vi "ChannelSettings.vi"() -> ()   [LabVIEW 2019]
uses:
  <vilib>/Bytelabs/ByteChannelsSetting/ChannelSettingsLib/ChannelsClasses/ChannelAnalog/AnalogRio/AnalogRio.lvclass
  C:/Program Files (x86)/National Instruments/LabVIEW 2019/vi.lib/Bytelabs/ByteChannelsSetting/ChannelSettingsLib/ChannelsClasses/ChannelAnalog/AnalogIn/AnalogIn.lvclass
  TypeDef/SubPanelType.ctl
  <vilib>/Bytelabs/ByteChannelsSetting/ChannelSettingsLib/ChannelsRepos/ChannelsRepoXML/ChannelsRepoXML.lvclass
  C:/Program Files (x86)/National Instruments/LabVIEW 2019/vi.lib/Bytelabs/ByteChannelsSetting/ChannelSettingsLib/ChannelsRepos/ChannelsRepoBase/ChannelsRepoBase.lvclass
  <vilib>/Bytelabs/ByteChannelsSetting/ChannelSettingsLib/ChannelsRepos/ChannelsRepoBase/ShowCreateUI.vi
  <vilib>/Bytelabs/ByteChannelsSetting/ChannelSettingsLib/ChannelsRepos/ChannelsRepoBase/ShowChannelConfiguration.vi
  <vilib>/Bytelabs/ByteChannelsSetting/ChannelSettingsLib/ChannelsRepos/ChannelsRepoBase/ChannelsRepoBase.lvclass
  <vilib>/Bytelabs/ByteSimpleQ/ByteSimpleQ/ByteSimpleQ.lvlib
panel:
  in  "Tree":string(tree)
  in  "Create":bool caption="Add Row"
  in  "Delete":bool caption="Delete Row"
  in  "Exit":bool
  in  "Apply":bool
  # "CHANNEL SETTING"
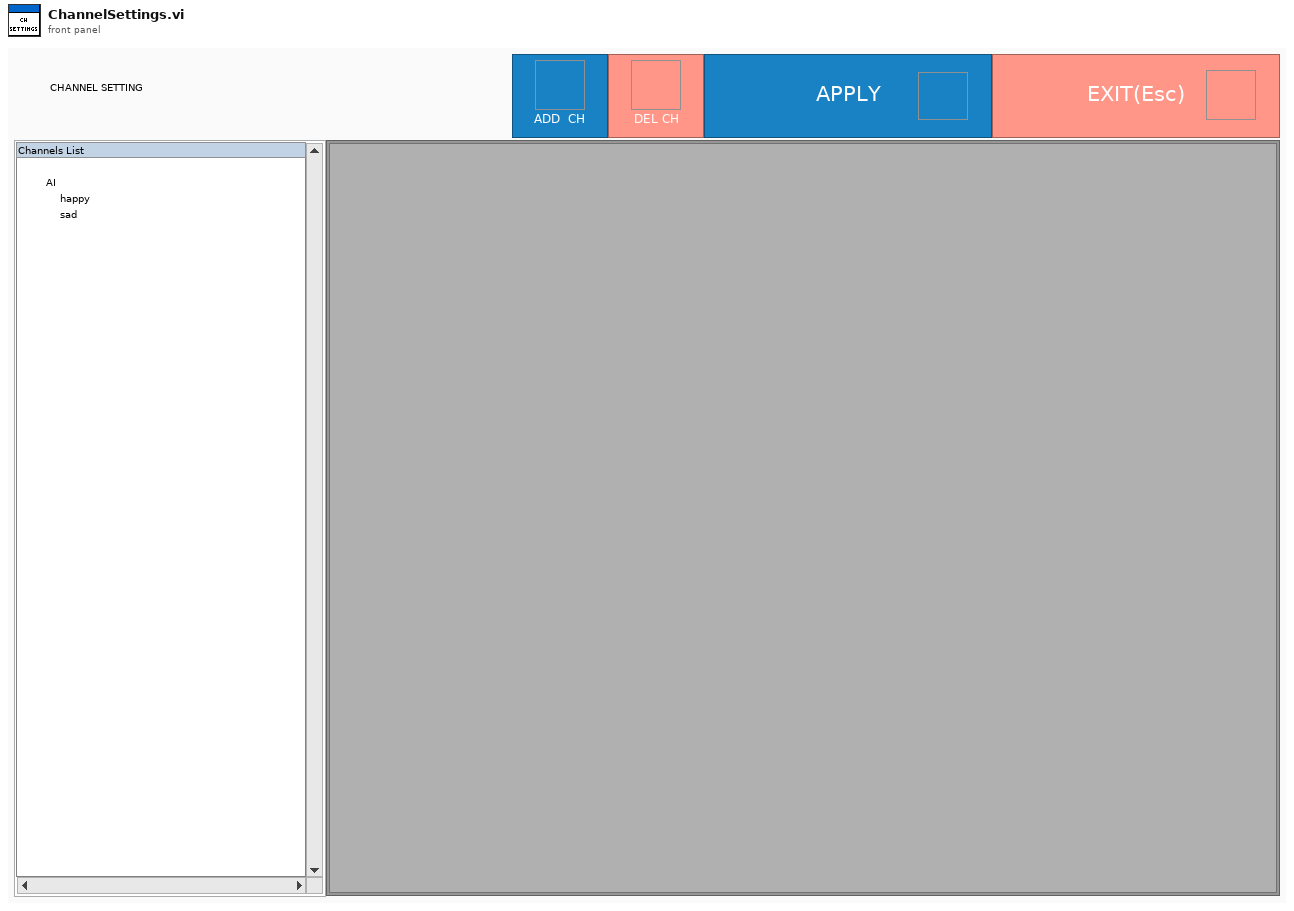
[diagram p1: front panel]
types:
  T1 = enum8{"Enabled", "Disabled", "Disabled and Grayed Out"}
  T2 = cluster{"queue out":refnum<queue>, "ChannelsRepoBase out":refnum<class "ChannelsRepoXML.lvclass">, "Close Event":refnum<user-event>, "Modify Ref":refnum<vi>, "Create Ref":refnum<vi>, "Mode":string, "Tree":refnum<vi>, "Tag":string, "ChannelsRepoBase out":refnum<class "ChannelsRepoXML.lvclass">}
  T3 = typedef "SubPanelType.ctl" = cluster{"Modality":string, "Tag":string}
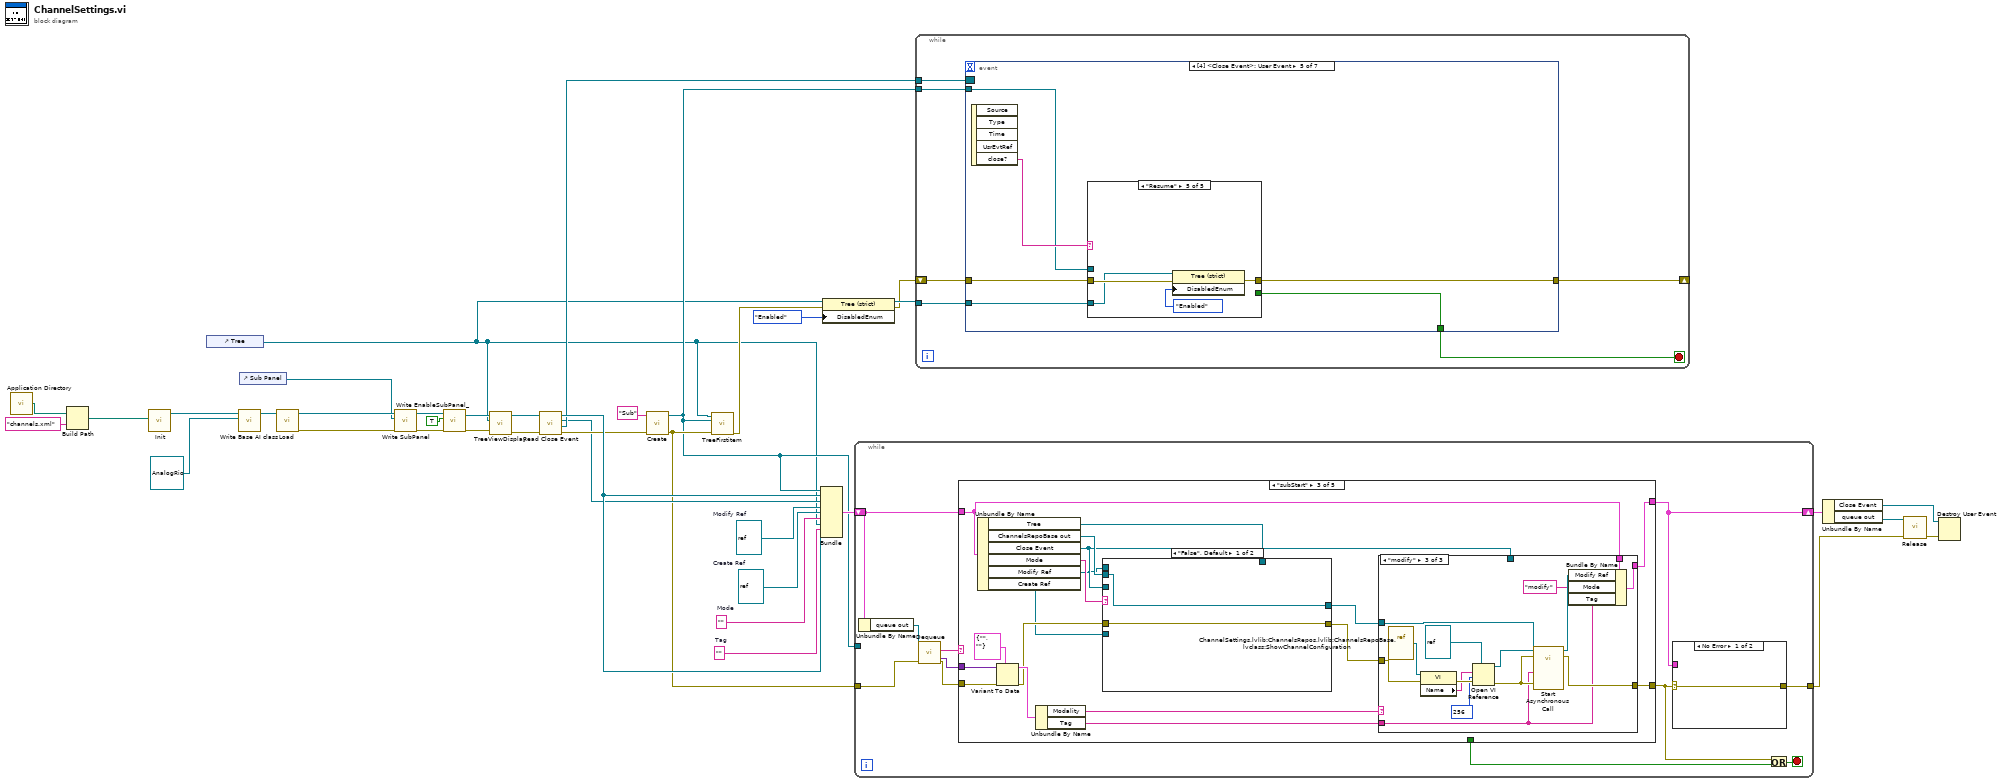
[diagram p0: block diagram]
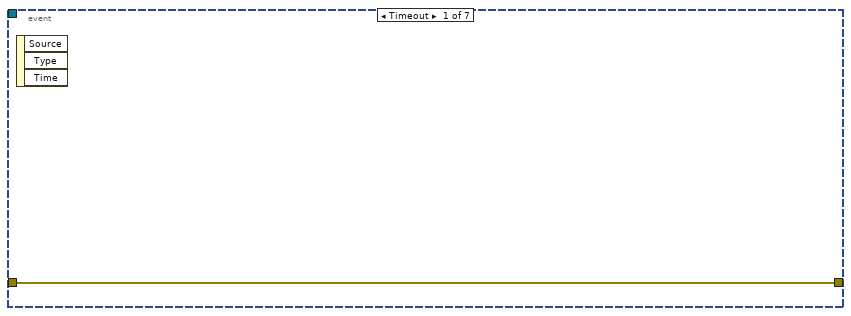
[diagram p2: hidden frame]
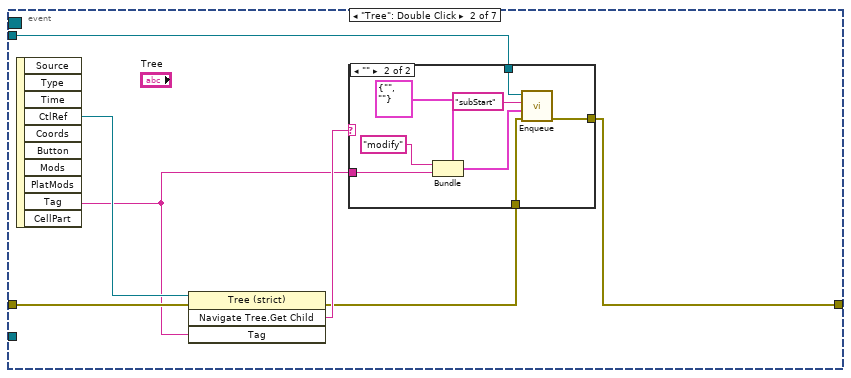
[diagram p3: hidden frame]
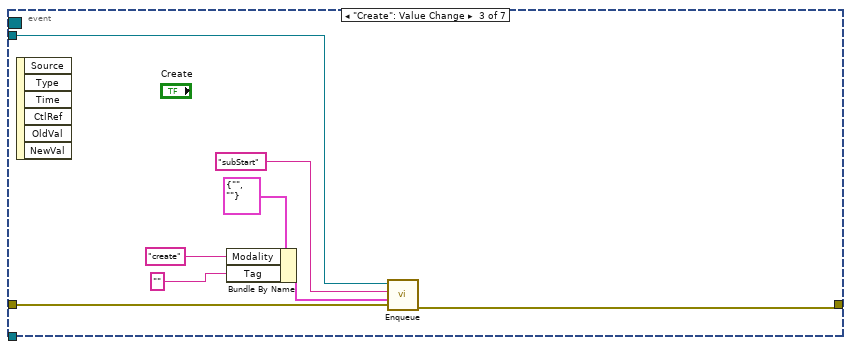
[diagram p5: hidden frame]
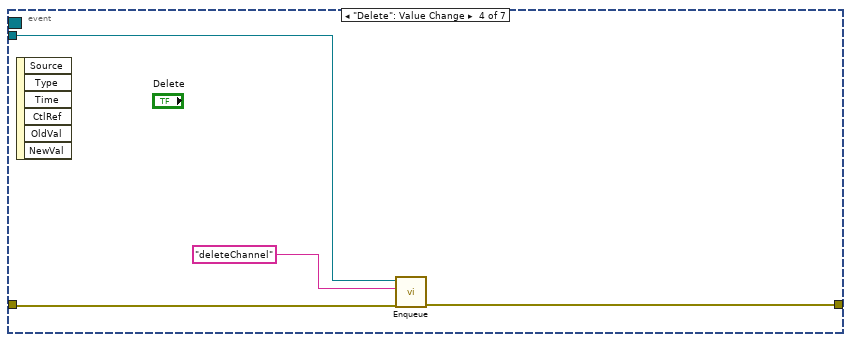
[diagram p6: hidden frame]
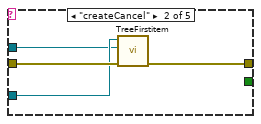
[diagram p8: hidden frame]
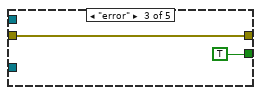
[diagram p9: hidden frame]
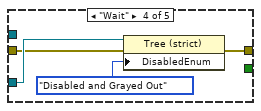
[diagram p10: hidden frame]
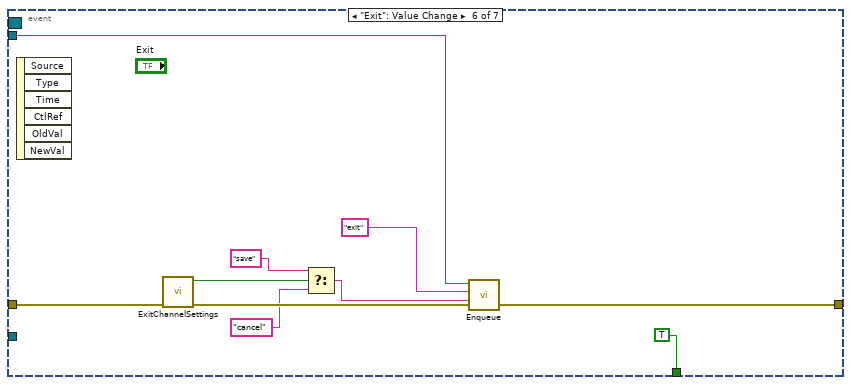
[diagram p11: hidden frame]
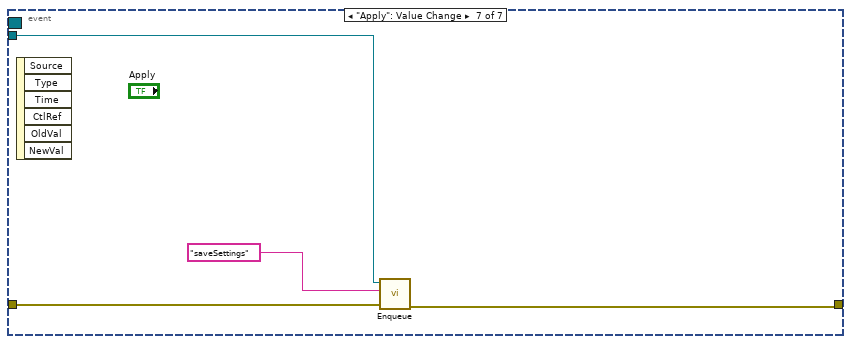
[diagram p12: hidden frame]
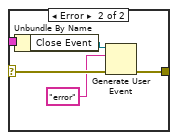
[diagram p13: hidden frame]
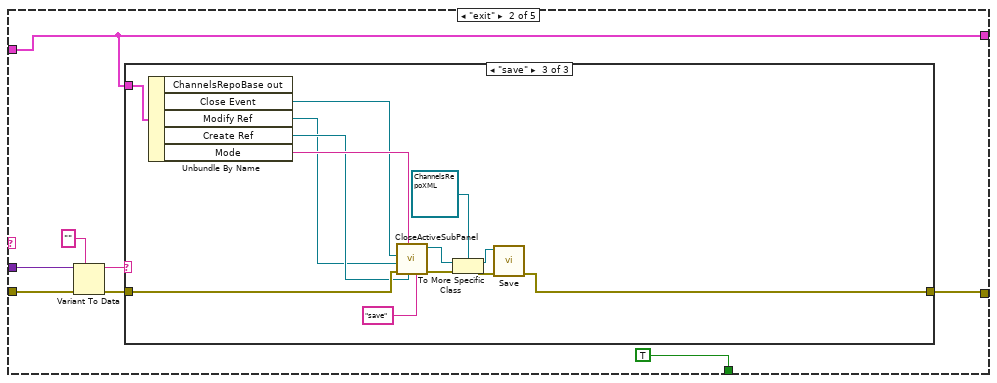
[diagram p15: hidden frame]
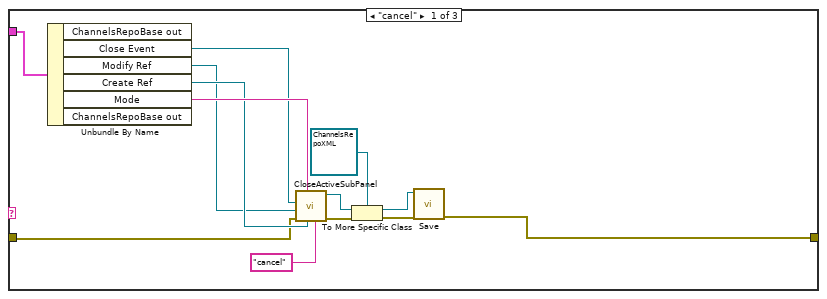
[diagram p16: hidden frame]
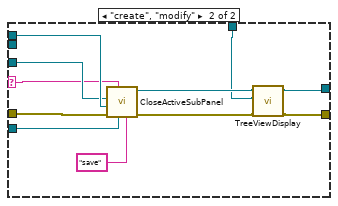
[diagram p18: hidden frame]
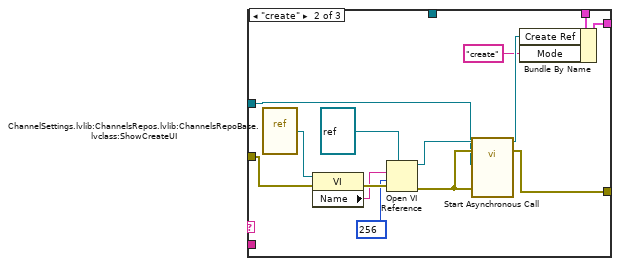
[diagram p20: hidden frame]
diagram:
  w29 = ""  # Tag
  w33 = refnum<vi> refnum  # Create Ref
  w34 = refnum<vi> refnum  # Modify Ref
  w32 = ""  # Mode
  n1 = call <vilib>:"Application Directory.vi"() -> ("Application Directory"=w18:path)
  n2 = Build Path(base path=w18, name or relative path="channels.xml") -> (appended path=w16:path)
  n3 = call <vilib>:"Init.vi"("XML file path"=w16) -> ("ChannelsRepoXML out"=w17:refnum<class "ChannelsRepoXML.lvclass">)  [unwired: 10 in]
  n4 = control-ref of="Tree"() -> (w5:refnum<vi>)
  n5 = call-dynamic "Write Base AI class.vi"("ChannelsClasses.lvlib:AnalogIn.lvclass"=refnum<class "AnalogRio.lvclass"> refnum ("ChannelSettings.lvlib:ChannelsClasses.lvlib:AnalogRio.lvclass"), "ChannelsRepoBase in"=w17) -> ("ChannelsRepoBase out"=w11:refnum<class "ChannelsRepoXML.lvclass">)  [unwired: 9 in]
  n6 = control-ref of="Sub Panel"() -> (w1:refnum<vi>)
  n7 = call <vilib>:"Load.vi"("ChannelsRepoBase in"=w11) -> ("error out"=w3:errorcluster, "ChannelsRepoBase out"=w35:refnum<class "ChannelsRepoXML.lvclass">)  [unwired: 8 in, 1 out]
  n8 = call-dynamic "Write SubPanel.vi"("error in (no error)"=w3, "SubPanel"=w1, "ChannelsRepoBase in"=w35) -> ("error out"=w38:errorcluster, "ChannelsRepoBase out"=w37:refnum<class "ChannelsRepoXML.lvclass">)  [unwired: 7 in]
  n9 = call-dynamic "Write EnableSubPanel_.vi"("error in (no error)"=w38, "EnableSubPanel?"=TRUE, "ChannelsRepoBase in"=w37) -> ("error out"=w15:errorcluster, "ChannelsRepoBase out"=w12:refnum<class "ChannelsRepoXML.lvclass">)  [unwired: 7 in]
  n10 = call-dynamic "TreeViewDisplay.vi"("error in (no error)"=w15, "Tree ref"=w5, "ChannelsRepoBase in"=w12) -> ("error out"=w14:errorcluster, "ChannelsRepoBase out"=w13:refnum<class "ChannelsRepoXML.lvclass">)  [unwired: 7 in]
  n11 = call-dynamic "Read Close Event.vi"("error in (no error)"=w14, "ChannelsRepoBase in"=w13) -> ("error out"=w22:errorcluster, "Event Refnum"=w21:refnum<event-registration>, "Close Event"=w20:refnum<user-event>, "ChannelsRepoBase out"=w23:refnum<class "ChannelsRepoXML.lvclass">)  [unwired: 6 in]
  n12 = call <vilib>:"Create.vi"("error in (no error)"=w22, "name (unnamed)"="Sub") -> ("error out"=w10:errorcluster, "queue out"=w9:refnum<queue>)  [unwired: 7 in, 1 out]
  n13 = call <vilib>:"TreeFirstitem.vi"("error in (no error)"=w10, "queue in"=w9, "TreeControl in"=w5) -> ("error out"=w7:errorcluster)  [unwired: 8 in]
  n14 = Bundle("queue out"=w9, "ChannelsRepoBase out"=w23, "Close Event"=w20, "Modify Ref"=w34, "Create Ref"=w33, "Mode"=w32, "Tree"=w5, "Tag"=w29, "ChannelsRepoBase out"=w23) -> (w31:T2)  [unwired: 1 in]
  n15 = property class="Tree (strict)"(reference=w5, error in=w7, "DisabledEnum"=T1."Enabled" ("Disabled")) -> (reference out=w6:refnum<vi>, error out=w4:errorcluster)
  n16 = while {
    tunnel: w9 -> [_]
    shift-right: [w41] -> w28
    shift-left: w31 -> [w40]
    tunnel: w10 -> [w49]
    tunnel: [w45] -> w26
    stop <- w44 stop-if-true
    n17 = Unbundle By Name(w40) -> ("queue out"=w39:refnum<queue>)
    n18 = call <vilib>:"Dequeue.vi"("error in (no error)"=w49, "queue in"=w39) -> ("error out"=w46:errorcluster, "data"=w47:variant, "message"=w48:string)  [unwired: 5 in, 2 out]
    n19 = case shown="\"subStart\"" w48 {
      tunnel: w47 -> [_ w63 w109 _ _]
      tunnel: w46 -> [w57 w64 w110 w166 w219]
      tunnel: w40 -> [w56 w58 w108 w157 w220]
      tunnel: [w57 w59 w106 w164 w213] -> w42
      tunnel: [w56 w58 w107 w156 w212] -> w41
      tunnel: [_ TRUE _ _ _] -> w43
      frame Default {
      }
      frame "exit" {
        n20 = Variant To Data(error in=w64, type="" ("message"), Variant=w63) -> (data=w61:string, error out=w60:errorcluster)
        n21 = case shown="\"save\"" w61 {
          tunnel: w60 -> [w70 w79 w88]
          tunnel: [w67 w79 w81] -> w59
          tunnel: w58 -> [w71 _ w89]
          frame "cancel" {
            n22 = Unbundle By Name(w71) -> ("Close Event"=w74:refnum<user-event>, "Modify Ref"=w72:refnum<vi>, "Create Ref"=w73:refnum<vi>, "Mode"=w75:string)  [unwired: 2 out]
            n23 = call <vilib>:"CloseActiveSubPanel.vi"("Save?"="cancel", "Create Ref"=w73, "Mode"=w75, "error in (no error)"=w70, "Modify Ref"=w72, "close?"=w74) -> ("error out"=w77:errorcluster, "ChannelsRepoBase out"=w76:refnum<class "ChannelsRepoXML.lvclass">)  [unwired: 3 in, 1 out]
            n24 = To More Specific Class(target class=refnum<class "ChannelsRepoXML.lvclass"> refnum ("ChannelsRepoBase out"), reference=w76, error in=w77) -> (specific class reference=w66:refnum<class "ChannelsRepoXML.lvclass">, error out=w68:errorcluster)
            n25 = call-dynamic "Save.vi"("error in (no error)"=w68, "ChannelsRepoXML in"=w66) -> ("error out"=w67:errorcluster)  [unwired: 8 in, 1 out]
          }
          frame Default {
          }
          frame "save" {
            n26 = Unbundle By Name(w89) -> ("Close Event"=w86:refnum<user-event>, "Modify Ref"=w84:refnum<vi>, "Create Ref"=w85:refnum<vi>, "Mode"=w87:string)  [unwired: 1 out]
            n27 = call <vilib>:"CloseActiveSubPanel.vi"("Save?"="save", "Create Ref"=w85, "Mode"=w87, "error in (no error)"=w88, "Modify Ref"=w84, "close?"=w86) -> ("error out"=w91:errorcluster, "ChannelsRepoBase out"=w90:refnum<class "ChannelsRepoXML.lvclass">)  [unwired: 3 in, 1 out]
            n28 = To More Specific Class(target class=refnum<class "ChannelsRepoXML.lvclass"> refnum ("ChannelsRepoBase out"), reference=w90, error in=w91) -> (specific class reference=w80:refnum<class "ChannelsRepoXML.lvclass">, error out=w82:errorcluster)
            n29 = call-dynamic "Save.vi"("error in (no error)"=w82, "ChannelsRepoXML in"=w80) -> ("error out"=w81:errorcluster)  [unwired: 8 in, 1 out]
          }
        }
      }
      frame "subStart" {
        n30 = Unbundle By Name(w108) -> ("Tree"=w93:refnum<vi>, "ChannelsRepoBase out"=w99:refnum<class "ChannelsRepoXML.lvclass">, "Close Event"=w97:refnum<user-event>, "Mode"=w100:string, "Modify Ref"=w96:refnum<vi>, "Create Ref"=w95:refnum<vi>)
        n31 = Variant To Data(error in=w110, type=T3 {"Modality"="", "Tag"=""}, Variant=w109) -> (data=w105:T3, error out=w103:errorcluster)
        n32 = Unbundle By Name(w105) -> ("Modality"=w94:string, "Tag"=w102:string)
        n33 = case shown="\"False\", Default" w100 {
          selector: w100 -> [_ w118]
          tunnel: w103 -> [w112 w123]
          tunnel: [w112 w114] -> w101
          tunnel: w99 -> [w111 _]
          tunnel: [w111 w117] -> w98
          tunnel: w97 -> [_ w119]
          tunnel: w96 -> [_ w120]
          tunnel: w95 -> [_ w121]
          tunnel: w93 -> [_ w113]
          frame "False", Default {
          }
          frame "create", "modify" {
            n34 = call <vilib>:"CloseActiveSubPanel.vi"("Save?"="save", "Create Ref"=w121, "Mode"=w118, "error in (no error)"=w123, "Modify Ref"=w120, "close?"=w119) -> ("error out"=w115:errorcluster, "ChannelsRepoBase out"=w116:refnum<class "ChannelsRepoXML.lvclass">)  [unwired: 3 in, 1 out]
            n35 = call-dynamic "TreeViewDisplay.vi"("error in (no error)"=w115, "Tree ref"=w113, "ChannelsRepoBase in"=w116) -> ("error out"=w114:errorcluster, "ChannelsRepoBase out"=w117:refnum<class "ChannelsRepoXML.lvclass">)  [unwired: 7 in]
          }
        }
        n36 = case shown="\"modify\"" w94 {
          tunnel: w108 -> [w124 w130 w147]
          tunnel: [w124 w129 w144] -> w107
          tunnel: [w125 w128 w143] -> w106
          tunnel: w97 -> [_ _ _]
          tunnel: w101 -> [w125 w127 w142]
          tunnel: w98 -> [_ w126 w140]
          tunnel: w102 -> [_ _ w141]
          frame Default {
          }
          frame "create" {
            n37 = vi-ref "ChannelSettings.lvlib:ChannelsRepos.lvlib:ChannelsRepoBase.lvclass:ShowCreateUI.vi"() -> (w139:refnum<vi>)
            n38 = property class="VI"(reference=w139, error in=w127) -> (error out=w138:errorcluster, "Name"=w137:string)  [unwired: 1 out]
            n39 = Open VI Reference(type specifier VI Refnum (for type only)=refnum<vi> refnum, vi path=w137, options=256, error in (no error)=w138) -> (vi reference=w134:refnum<vi>, error out=w133:errorcluster)  [unwired: 2 in]
            n40 = call-by-ref "Start Asynchronous Call"(reference=w134, error in=w133, 8:"error in (no error)"=w133, "ChannelBase in"=w126) -> (reference out=w132:refnum<vi>, error out=w128:errorcluster)  [unwired: 7 in, 3 out]
            n41 = Bundle By Name(cluster=w130, "Create Ref"=w132, "Mode"="create") -> (w129:T2)
          }
          frame "modify" {
            n42 = vi-ref "ChannelSettings.lvlib:ChannelsRepos.lvlib:ChannelsRepoBase.lvclass:ShowChannelConfiguration.vi"() -> (w154:refnum<vi>)
            n43 = property class="VI"(reference=w154, error in=w142) -> (error out=w153:errorcluster, "Name"=w152:string)  [unwired: 1 out]
            n44 = Open VI Reference(type specifier VI Refnum (for type only)=refnum<vi> refnum, vi path=w152, options=256, error in (no error)=w153) -> (vi reference=w149:refnum<vi>, error out=w148:errorcluster)  [unwired: 2 in]
            n45 = call-by-ref "Start Asynchronous Call"(reference=w149, error in=w148, 8:"error in (no error)"=w148, "tag"=w141, "ChannelsRepoBase in"=w140) -> (reference out=w146:refnum<vi>, error out=w143:errorcluster)  [unwired: 6 in, 3 out]
            n46 = Bundle By Name(cluster=w147, "Modify Ref"=w146, "Mode"="modify", "Tag"=w141) -> (w144:T2)
          }
        }
      }
      frame "deleteChannel" {
        n47 = Unbundle By Name(w157) -> ("queue out"=w155:refnum<queue>, "ChannelsRepoBase out"=w167:refnum<class "ChannelsRepoXML.lvclass">, "Close Event"=w165:refnum<user-event>, "Mode"=w161:string, "Modify Ref"=w160:refnum<vi>, "Create Ref"=w159:refnum<vi>, "Tree"=w158:refnum<vi>)  [unwired: 1 out]
        n48 = call <vilib>:"DeleteChannelConfirmation.vi"("error in (no error)"=w166) -> ("error out"=w162:errorcluster, "Confirmed"=w163:bool)  [unwired: 9 in]
        n49 = case shown="True" w163 {
          tunnel: w167 -> [_ _]
          tunnel: w165 -> [_ w186]
          tunnel: [w169 w179] -> w164
          tunnel: w162 -> [w169 w190]
          tunnel: w161 -> [_ w189]
          tunnel: w160 -> [_ w188]
          tunnel: w159 -> [_ w187]
          tunnel: w158 -> [_ w170]
          tunnel: w157 -> [w168 w183]
          tunnel: [w168 w182] -> w156
          tunnel: w155 -> [_ w178]
          frame False {
          }
          frame True {
            n50 = call <vilib>:"CloseActiveSubPanel.vi"("Save?"="cancel", "Create Ref"=w187, "Mode"=w189, "error in (no error)"=w190, "Modify Ref"=w188, "close?"=w186) -> ("error out"=w191:errorcluster, "Tag"=w184:string, "ChannelsRepoBase out"=w175:refnum<class "ChannelsRepoXML.lvclass">)  [unwired: 3 in]
            n51 = call <vilib>:"DeleteChannel.vi"("error in (no error)"=w191, "tag"=w184, "ChannelsRepoBase in"=w175) -> ("error out"=w173:errorcluster, "ChannelsRepoBase out"=w174:refnum<class "ChannelsRepoXML.lvclass">)  [unwired: 6 in, 1 out]
            n52 = call-dynamic "TreeViewDisplay.vi"("error in (no error)"=w173, "Tree ref"=w170, "ChannelsRepoBase in"=w174) -> ("error out"=w172:errorcluster, "ChannelsRepoBase out"=w171:refnum<class "ChannelsRepoXML.lvclass">)  [unwired: 7 in]
            n53 = To More Specific Class(target class=refnum<class "ChannelsRepoXML.lvclass"> refnum ("ChannelsRepoBase out"), reference=w171, error in=w172) -> (specific class reference=w177:refnum<class "ChannelsRepoXML.lvclass">, error out=w180:errorcluster)
            n54 = call <vilib>:"TreeFirstitem.vi"("error in (no error)"=w180, "queue in"=w178, "TreeControl in"=w170) -> ("error out"=w179:errorcluster)  [unwired: 8 in]
            n55 = Bundle By Name(cluster=w183, "ChannelsRepoBase out"=w177, "Mode"="") -> (w182:T2)
          }
        }
      }
      frame "saveSettings" {
        n56 = Unbundle By Name(w220) -> ("Tree"=w194:refnum<vi>, "Close Event"=w198:refnum<user-event>, "Modify Ref"=w217:refnum<vi>, "Create Ref"=w216:refnum<vi>, "Mode"=w215:string)  [unwired: 1 out]
        n57 = call <vilib>:"CloseActiveSubPanel.vi"("Save?"="save", "Create Ref"=w216, "Mode"=w215, "error in (no error)"=w219, "Modify Ref"=w217, "close?"=w198) -> ("error out"=w214:errorcluster, "Tag"=w210:string, "ChannelsRepoBase out"=w207:refnum<class "ChannelsRepoXML.lvclass">)  [unwired: 3 in]
        n58 = To More Specific Class(target class=refnum<class "ChannelsRepoXML.lvclass"> refnum ("ChannelsRepoBase out"), reference=w207, error in=w214) -> (specific class reference=w206:refnum<class "ChannelsRepoXML.lvclass">, error out=w209:errorcluster)
        n59 = call-dynamic "Save.vi"("error in (no error)"=w209, "ChannelsRepoXML in"=w206) -> ("error out"=w193:errorcluster, "ChannelsRepoXML out"=w196:refnum<class "ChannelsRepoXML.lvclass">)  [unwired: 8 in]
        n60 = call-dynamic "TreeViewDisplay.vi"("error in (no error)"=w193, "Tree ref"=w194, "ChannelsRepoBase in"=w196) -> ("error out"=w192:errorcluster, "ChannelsRepoBase out"=w195:refnum<class "ChannelsRepoXML.lvclass">)  [unwired: 7 in]
        n61 = vi-ref "ChannelSettings.lvlib:ChannelsRepos.lvlib:ChannelsRepoBase.lvclass:ShowChannelConfiguration.vi"() -> (w205:refnum<vi>)
        n62 = property class="VI"(reference=w205, error in=w192) -> (error out=w204:errorcluster, "Name"=w203:string)  [unwired: 1 out]
        n63 = Open VI Reference(type specifier VI Refnum (for type only)=refnum<vi> refnum, vi path=w203, options=256, error in (no error)=w204) -> (vi reference=w200:refnum<vi>, error out=w199:errorcluster)  [unwired: 2 in]
        n64 = call-by-ref "Start Asynchronous Call"(reference=w200, error in=w199, 8:"error in (no error)"=w199, "tag"=w210, "ChannelsRepoBase in"=w195) -> (reference out=w197:refnum<vi>, error out=w213:errorcluster)  [unwired: 6 in, 3 out]
        n65 = Bundle By Name(cluster=w220, "ChannelsRepoBase out"=w206, "ChannelsRepoBase out"=w195, "Modify Ref"=w197, "Mode"="modify", "Tag"=w210) -> (w212:T2)
      }
    }
    n66 = case shown="No Error" w42 {
      selector: w42 -> [w50 w54]
      tunnel: [w50 w53] -> w45
      tunnel: w41 -> [_ w55]
      frame No Error {
      }
      frame Error {
        n67 = Unbundle By Name(w55) -> ("Close Event"=w52:refnum<user-event>)
        n68 = Generate User Event(user event=w52, event data cluster="error" ("event data"), error in=w54) -> (error out=w53:errorcluster)  [unwired: 1 in, 1 out]
      }
    }
    n69 = Or(x=w42, y=w43) -> (x .or. y?=w44:bool)
  }
  n70 = while {
    tunnel: w9 -> [w225]
    shift-right: [w224] -> _
    shift-left: w4 -> [w226]
    tunnel: w21 -> [w222]
    tunnel: w6 -> [w221]
    stop <- w223 stop-if-true
    n71 = event shown="[4] <Close Event>: User Event" {
      selector: w222 -> [_ _ _ _ _ _ _]
      dyn-events: _ -> [_ _ _ _ _ _ _]
      timeout: _ -> [_ _ _ _ _ _ _]
      tunnel: w226 -> [w227 w233 w246 w254 w261 w282 w289]
      tunnel: w225 -> [_ w230 w244 w252 w258 w284 w287]
      tunnel: [w227 w229 w245 w253 w260 w285 w288] -> w224
      tunnel: [_ _ _ _ w256 TRUE _] -> w223
      tunnel: w221 -> [_ _ _ _ w257 _ _]
      event Timeout {
        n72 = event-data() -> ()  [unwired: 1 in, 3 out]
      }
      event "Tree": Double Click {
        n73 = event-data() -> ("CtlRef"=w232:refnum<vi>, "Tag"=w231:string)  [unwired: 1 in, 8 out]
        n74 = invoke class="Tree (strict)" method="Navigate Tree.Get Child"(reference=w232, error in=w233, "Tag"=w231) -> (error out=w228:errorcluster, "Navigate Tree:Get Child"=w234:string)  [unwired: 1 in, 2 out]
        n75 = case shown="\"\"" w234 {
          tunnel: [w235 w241] -> w229
          tunnel: w231 -> [_ w239]
          tunnel: w230 -> [_ w237]
          tunnel: w228 -> [w235 w236]
          frame Default {
          }
          frame "" {
            n76 = Bundle(cluster=T3 {"Modality"="", "Tag"=""}, "Modality"="modify", "Tag"=w239) -> (w242:T3)
            n77 = call <vilib>:"Enqueue.vi"("error in (no error)"=w236, "data"=w242, "message"="subStart", "queue in"=w237) -> ("error out"=w241:errorcluster)  [unwired: 5 in, 2 out]
          }
        }
      }
      event "Create": Value Change {
        n78 = event-data() -> ()  [unwired: 1 in, 6 out]
        n79 = Bundle By Name(cluster=T3 {"Modality"="", "Tag"=""}, "Modality"="create", "Tag"="") -> (w248:T3)
        n80 = call <vilib>:"Enqueue.vi"("error in (no error)"=w246, "data"=w248, "message"="subStart", "queue in"=w244) -> ("error out"=w245:errorcluster)  [unwired: 5 in, 2 out]
      }
      event "Delete": Value Change {
        n81 = event-data() -> ()  [unwired: 1 in, 6 out]
        n82 = call <vilib>:"Enqueue.vi"("error in (no error)"=w254, "message"="deleteChannel", "queue in"=w252) -> ("error out"=w253:errorcluster)  [unwired: 6 in, 2 out]
      }
      event User Event {
        n83 = event-data() -> ("close?"=w259:string)  [unwired: 1 in, 4 out]
        n84 = case shown="\"Resume\"" w259 {
          tunnel: w261 -> [w262 w266 w268 w270 w275]
          tunnel: [w262 w265 w268 w269 w274] -> w260
          tunnel: w258 -> [_ w263 _ _ _]
          tunnel: w257 -> [_ w264 _ w272 w273]
          tunnel: [_ _ TRUE _ _] -> w256
          frame Default {
          }
          frame "createCancel" {
            n85 = call <vilib>:"TreeFirstitem.vi"("error in (no error)"=w266, "queue in"=w263, "TreeControl in"=w264) -> ("error out"=w265:errorcluster)  [unwired: 8 in]
          }
          frame "error" {
          }
          frame "Wait" {
            n86 = property class="Tree (strict)"(reference=w272, error in=w270, "DisabledEnum"=T1."Disabled and Grayed Out" ("Disabled")) -> (error out=w269:errorcluster)  [unwired: 1 out]
          }
          frame "Resume" {
            n87 = property class="Tree (strict)"(reference=w273, error in=w275, "DisabledEnum"=T1."Enabled" ("Disabled")) -> (error out=w274:errorcluster)  [unwired: 1 out]
          }
        }
      }
      event "Exit": Value Change {
        n88 = event-data() -> ()  [unwired: 1 in, 6 out]
        n89 = call <vilib>:"ExitChannelSettings.vi"("error in (no error)"=w282) -> ("error out"=w281:errorcluster, "Confirmed"=w280:bool)  [unwired: 9 in]
        n90 = Select(t="save" ("message"), s=w280, f="cancel" ("message")) -> (s? t:f=w277:string)
        n91 = call <vilib>:"Enqueue.vi"("error in (no error)"=w281, "data"=w277, "message"="exit", "queue in"=w284) -> ("error out"=w285:errorcluster)  [unwired: 5 in, 2 out]
      }
      event "Apply": Value Change {
        n92 = event-data() -> ()  [unwired: 1 in, 6 out]
        n93 = call <vilib>:"Enqueue.vi"("error in (no error)"=w289, "message"="saveSettings", "queue in"=w287) -> ("error out"=w288:errorcluster)  [unwired: 6 in, 2 out]
      }
    }
  }
  n94 = Unbundle By Name(w28) -> ("Close Event"=w27:refnum<user-event>, "queue out"=w24:refnum<queue>)
  n95 = call <vilib>:"Release.vi"("error in (no error)"=w26, "queue in"=w24) -> ("error out"=w25:errorcluster)  [unwired: 9 in]
  n96 = Destroy User Event(user event=w27, error in=w25) -> ()  [unwired: 1 out]
